vi "WAM-DC-HealthCheck.vi"(6 "COMPORT":refnum<visa-resource-name>="COM4", 8 "error in (no error)":errorcluster, 10 "reference in":refnum<vi>, 11 "LVObjectRefNum in":refnum<vi>) -> (0 "error out":errorcluster, 2 "comport":refnum<visa-resource-name>="COM4", 3 "i_mon":string)   [LabVIEW 2018]
uses:
  Initialize References/Sequence Globals.vi
  Tetra_Globals.vi
panel:
  out "supp_path":path
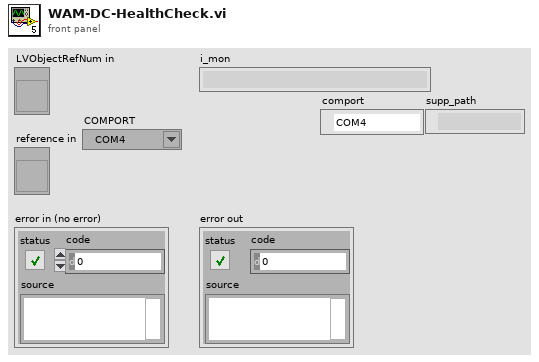
[diagram p1: front panel]
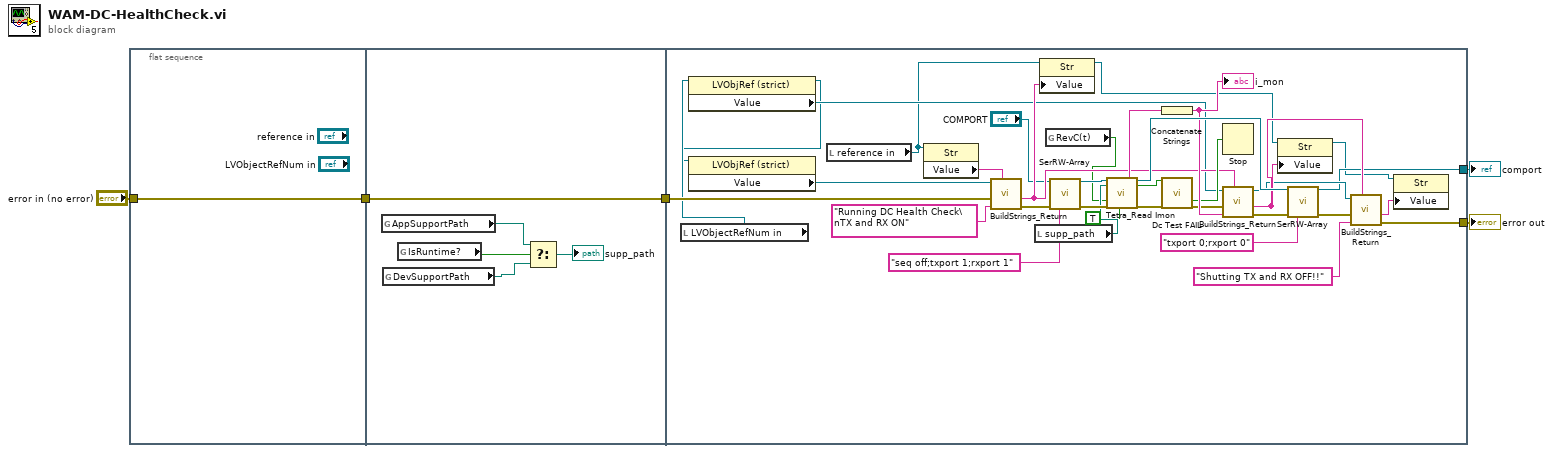
[diagram p0: block diagram]
diagram:
  n1 = flat-sequence {
    tunnel: "error in (no error)" -> [w6]
    tunnel: [w6] -> w1
    tunnel: [w11] -> w2
    tunnel: w1 -> [w11]
    tunnel: [w28] -> w4
    tunnel: [w20] -> w3
    tunnel: w2 -> [w46]
    frame #0 {
    }
    frame #1 {
      n2 = global read "Sequence Globals.vi" "AppSupportPath"() -> (w10:path)
      n3 = global read "Sequence Globals.vi" "DevSupportPath"() -> (w9:path)
      n4 = global read "Sequence Globals.vi" "IsRuntime?"() -> (w8:bool)
      n5 = Select(t=w10, s=w8, f=w9) -> (s? t:f=→"supp_path":path)
    }
    frame #2 {
      n6 = local read "LVObjectRefNum in"() -> (w16:refnum<vi>)
      n7 = property class="LVObjRef (strict)"(reference=w16) -> (reference out=w15:refnum<vi>, "Value"=w26:refnum<vi>)  [unwired: 1 in, 1 out]
      n8 = property class="LVObjRef (strict)"(reference=w15) -> ("Value"=w45:refnum<vi>)  [unwired: 1 in, 2 out]
      n9 = local read "reference in"() -> (w19:refnum<vi>)
      n10 = property class="Str"(reference=w19) -> ("Value"=w44:string)  [unwired: 1 in, 2 out]
      n11 = call "BuildStrings_Return.vi"("Input String"=w44, "New String"="Running DC Health Check\nTX and RX ON", "error in (no error)"=w46, "reference"=w45) -> ("error out"=w42:errorcluster, "concatenated string"=w29:string)  [unwired: 5 in, 1 out]
      n12 = local read "supp_path"() -> (w14:path)
      n13 = property class="Str"(reference=w19, "Value"=w29) -> (reference out=w18:refnum<vi>)  [unwired: 1 in, 1 out]
      n14 = global read "Tetra_Globals.vi" "RevC(t)"() -> (w13:bool)
      n15 = call "SerRW-Array.vi"("COMPORT"="COMPORT", "error in (no error)"=w42, "Command ( ; seperation)"="seq off;txport 1;rxport 1") -> ("comport"=w40:refnum<visa-resource-name>, "error out"=w39:errorcluster)  [unwired: 6 in, 5 out]
      n16 = call "Tetra_Read Imon.vi"("COMPORT"=w40, "ini limits directory (if blank will skip)"=w14, "rev_c(t)"=w13, "error in (no error)"=w39, "Meas_Limits"=TRUE) -> ("Result  0|1[PASS/FAIL]: dcv(7b) dci(7b)"=w38:string, "comport"=w37:refnum<visa-resource-name>, "Fail?(t)"=w30:bool, "error out"=w33:errorcluster)  [unwired: 9 in, 2 out]
      n17 = Concatenate Strings(w38) -> (w34:string)
      "i_mon" <- w34
      n18 = call "Dc Test FAIL"("Enable"=w30, "error in (no error)"=w33) -> ("Abort"=w31:bool, "error out"=w32:errorcluster)  [unwired: 16 in]
      n19 = Stop(stop? (T)=w31) -> ()
      n20 = call "BuildStrings_Return.vi"("Input String"=w29, "New String"=w34, "error in (no error)"=w32, "reference"=w26) -> ("error out"=w35:errorcluster, "concatenated string"=w25:string, "reference out"=w23:refnum<vi>)  [unwired: 5 in]
      n21 = property class="Str"(reference=w18, "Value"=w25) -> (reference out=w17:refnum<vi>)  [unwired: 1 in, 1 out]
      n22 = call "SerRW-Array.vi"("COMPORT"=w37, "error in (no error)"=w35, "Command ( ; seperation)"="txport 0;rxport 0") -> ("comport"=w20:refnum<visa-resource-name>, "error out"=w27:errorcluster)  [unwired: 6 in, 5 out]
      n23 = call "BuildStrings_Return.vi"("Input String"=w25, "New String"="Shutting TX and RX OFF!!", "error in (no error)"=w27, "reference"=w23) -> ("error out"=w28:errorcluster, "concatenated string"=w24:string)  [unwired: 5 in, 1 out]
      n24 = property class="Str"(reference=w17, "Value"=w24) -> ()  [unwired: 1 in, 2 out]
    }
  }
  "error out" <- w4
  "comport" <- w3
